vi "FP_SetAppearance.vi"(8 "error in (no error)":errorcluster, 9 "Front Panel Window:Window Bounds 2":T1={"Left"=0, "Top"=0, "Right"=800, "Bottom"=425}, 10 "Front Panel Window:Title":string="TCPMSG", 11 "vi path":path) -> (0 "error out":errorcluster)   [LabVIEW 2012, in "FP_FrontPanel.lvlib"]
uses:
  FP_FrontPanel.lvlib
  <vilib>/Utility/miscctls.llb/LVRectTypeDef.ctl
  <vilib>/Utility/miscctls.llb/LVPointTypeDef.ctl
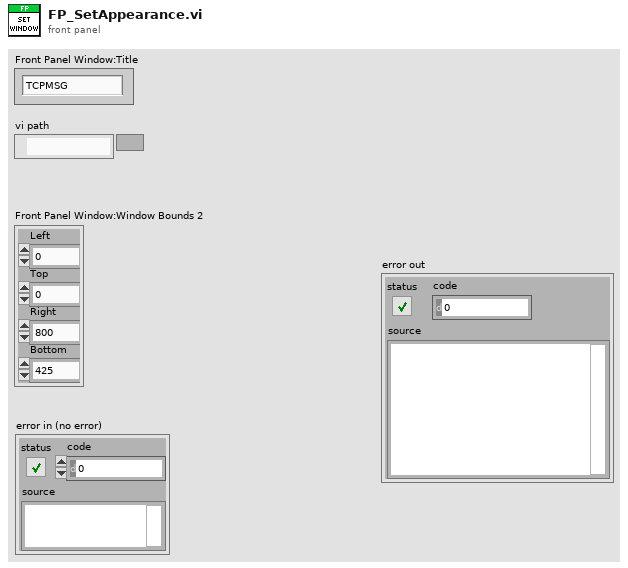
[diagram p1: front panel]
types:
  T1 = typedef "LVRectTypeDef.ctl" = cluster{"Left":i16, "Top":i16, "Right":i16, "Bottom":i16}
  T2 = typedef "LVPointTypeDef.ctl" = cluster{"Horizontal":i16, "Vertical":i16}
  T3 = enum32{"Invalid", "Standard", "Closed", "Hidden", "Minimized", "Maximized"}
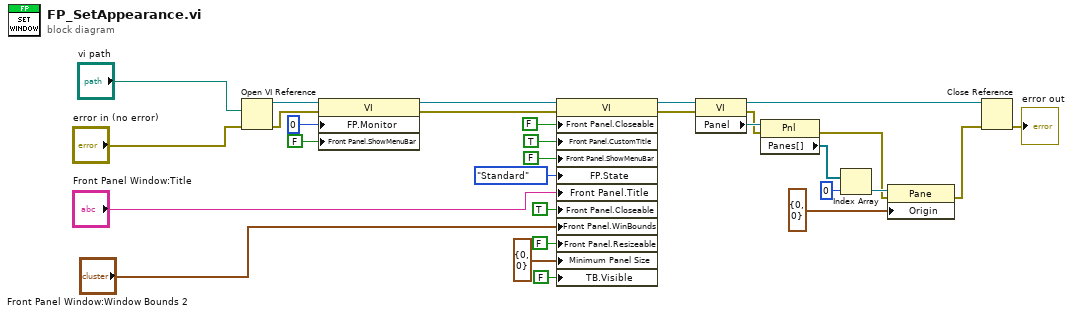
[diagram p0: block diagram]
diagram:
  n1 = Open VI Reference(vi path="vi path", error in (no error)="error in (no error)") -> (vi reference=w6:refnum<vi>, error out=w5:errorcluster)  [unwired: 4 in]
  n2 = property class="VI"(reference=w6, error in=w5, "FP.Monitor"=u16 0 ("Front Panel Window:Monitor"), "Front Panel.ShowMenuBar"=FALSE ("Front Panel Window:Show Menu Bar")) -> (reference out=w7:refnum<vi>, error out=w8:errorcluster)
  n3 = property class="VI"(reference=w7, error in=w8, "Front Panel.Closeable"=FALSE ("Front Panel Window:Closeable"), "Front Panel.CustomTitle"=TRUE ("Front Panel Window:Custom Title"), "Front Panel.ShowMenuBar"=FALSE ("Front Panel Window:Show Menu Bar"), "FP.State"=T3."Standard" ("Front Panel Window:State"), "Front Panel.Title"="Front Panel Window:Title", "Front Panel.Closeable"=TRUE ("Front Panel Window:Closeable"), "Front Panel.WinBounds"="Front Panel Window:Window Bounds 2", "Front Panel.Resizeable"=FALSE ("Front Panel Window:Resizable"), "Minimum Panel Size"=T2 {"Horizontal"=0, "Vertical"=0} ("Front Panel Window:Minimum Size"), "TB.Visible"=FALSE ("Tool Bar:Visible")) -> (reference out=w21:refnum<vi>, error out=w20:errorcluster)
  n4 = property class="VI"(reference=w21, error in=w20) -> (reference out=w12:refnum<vi>, error out=w18:errorcluster, "Panel"=w19:refnum<vi>)
  n5 = property class="Pnl"(reference=w19, error in=w18) -> (error out=w11:errorcluster, "Panes[]"=w17:refnum<vi>[])  [unwired: 1 out]
  n6 = Index Array(array=w17, index=0) -> (element=w16:refnum<vi>)
  n7 = property class="Pane"(reference=w16, error in=w11, "Origin"=T2 {"Horizontal"=0, "Vertical"=0}) -> (error out=w13:errorcluster)  [unwired: 1 out]
  n8 = Close Reference(reference=w12, error in (no error)=w13) -> (error out=→"error out":errorcluster)
